vi "JKISM++ Running Log - DebugTool.vi"() -> ()   [LabVIEW 2014]
uses:
  _Support/Typedef/_JKISM_GlobalLog_MSG.ctl
  _Support/Typedef/_JKISM_GlobalLog_MSG_TYPE.ctl
  _Support/GlobalEvent/FGV-GlobalEventRef.vi
  JKI State Machine++.lvlib
panel:
  out "State History":string
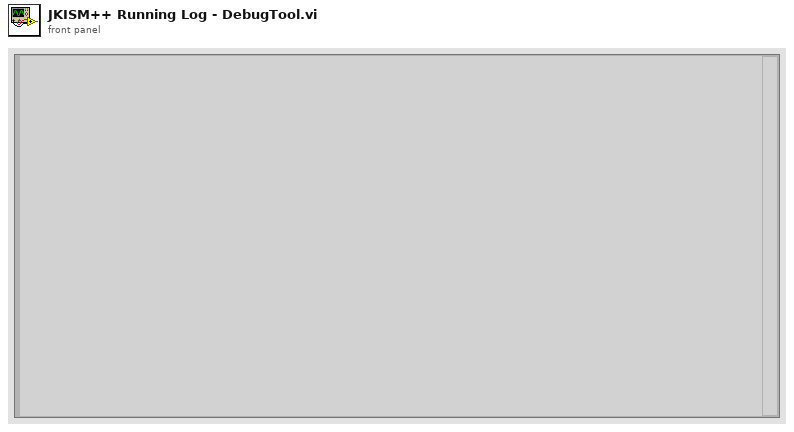
[diagram p1: front panel]
types:
  T1 = typedef "JKI State Machine++.lvlib/_JKISM_GlobalLog_MSG.ctl" = cluster{"Name(\"\" to use uuid)":string, "Current State":string, "Arguments":string, "Argument - State":string, "From Who":string, "Complete(T)/Start(F)":bool, "Type":T2}
  T2 = typedef "JKI State Machine++.lvlib/_JKISM_GlobalLog_MSG_TYPE.ctl" = enum16{"User Log", "State Change", "Status Change", "Interrupt Change", "Register", "Unregister"}
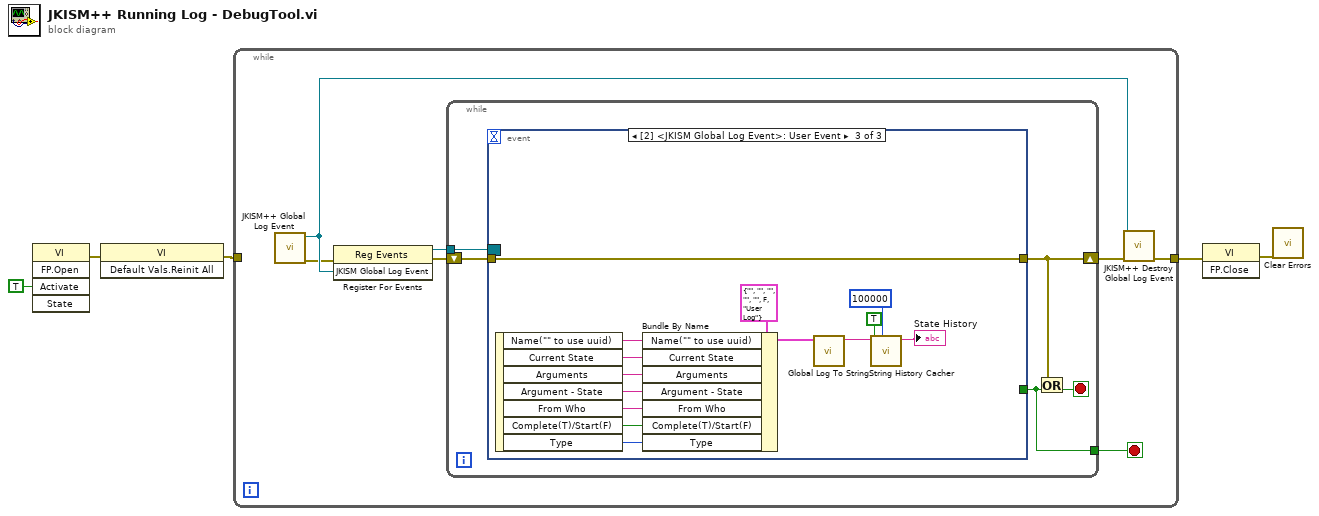
[diagram p0: block diagram]
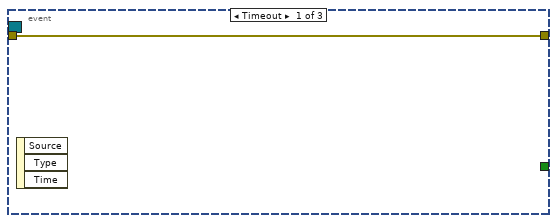
[diagram p2: hidden frame]
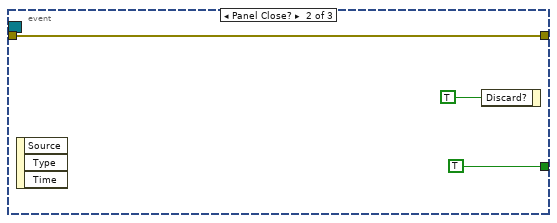
[diagram p3: hidden frame]
diagram:
  n1 = invoke class="VI" method="FP.Open"("Activate"=TRUE ("Activate?")) -> (error out=w4:errorcluster)  [unwired: 4 in, 4 out]
  n2 = invoke class="VI" method="Default Vals.Reinit All"(error in=w4) -> (error out=w3:errorcluster)  [unwired: 2 in, 2 out]
  n3 = while {
    tunnel: w3 -> [_]
    tunnel: [w6] -> w2
    stop <- w7 stop-if-true
    n4 = call "JKISM++ Global Log Event.vi"() -> ("Error out"=w8:errorcluster, "JKISM Global Log Event"=w9:refnum<user-event>)  [unwired: 10 in]
    n5 = register-events(error in=w8, w9) -> (reference out=w12:refnum<event-registration>, error out=w11:errorcluster)  [unwired: 1 in]
    n6 = while {
      tunnel: w12 -> [w17]
      shift-right: [w14] -> w10
      shift-left: w11 -> [w16]
      tunnel: [w13] -> w7
      stop <- w15 stop-if-true
      n7 = event shown="[2] <JKISM Global Log Event>: User Event" {
        selector: w17 -> [_ _ _]
        dyn-events: _ -> [_ _ _]
        timeout: _ -> [_ _ _]
        tunnel: w16 -> [w18 w21 w35]
        tunnel: [w18 w21 w35] -> w14
        tunnel: [_ TRUE ("Discard?") _] -> w13
        event Timeout {
          n8 = event-data() -> ()  [unwired: 1 in, 3 out]
        }
        event Panel Close? {
          n9 = event-data() -> ()  [unwired: 1 in, 3 out]
          n10 = event-data("Discard?"=TRUE) -> ()  [unwired: 1 in, 1 out]
        }
        event User Event {
          n11 = event-data() -> ("Name(\"\" to use uuid)"=w28:string, "Current State"=w27:string, "Arguments"=w26:string, "Argument - State"=w25:string, "From Who"=w24:string, "Complete(T)/Start(F)"=w23:bool, "Type"=w22:T2)  [unwired: 1 in]
          n12 = Bundle By Name(cluster=T1 {"Name(\"\" to use uuid)"="", "Current State"="", "Arguments"="", "Argument - State"="", "From Who"="", "Complete(T)/Start(F)"=FALSE, "Type"=enum."User Log"} ("Log"), "Name(\"\" to use uuid)"=w28, "Current State"=w27, "Arguments"=w26, "Argument - State"=w25, "From Who"=w24, "Complete(T)/Start(F)"=w23, "Type"=w22) -> (w29:T1)
          n13 = call "Global Log To String.vi"("Log"=w29) -> ("String"=w31:string)  [unwired: 9 in]
          n14 = call "String History Cacher.vi"("length"=100000, "Include Timestamp(T)"=TRUE ("Include Timestamp(F)"), "String"=w31) -> ("String Cache"=→"State History":string)  [unwired: 8 in]
        }
      }
      n15 = Or(x=w14, y=w13) -> (x .or. y?=w15:bool)
    }
    n16 = call "JKISM++ Destroy Global Log Event.vi"("Error in"=w10, "JKISM Global Log Event"=w9) -> ("Error out"=w6:errorcluster)  [unwired: 9 in]
  }
  n17 = invoke class="VI" method="FP.Close"(error in=w2) -> (error out=w1:errorcluster)  [unwired: 2 in, 2 out]
  n18 = call <vilib>:"Clear Errors.vi"("error in (no error)"=w1) -> ()  [unwired: 5 in, 2 out]
